vi "Read.vi"(8 "error in (no error)":errorcluster, 11 "DAQmx AI in":refnum<class "DAQmx AI.lvclass">) -> (0 "error out":errorcluster, 2 "Output":variant, 3 "DAQmx AI out":refnum<class "DAQmx AI.lvclass">)   [LabVIEW 2017, in "DAQmx AI.lvclass"]
uses:
  DAQmx AI.lvclass
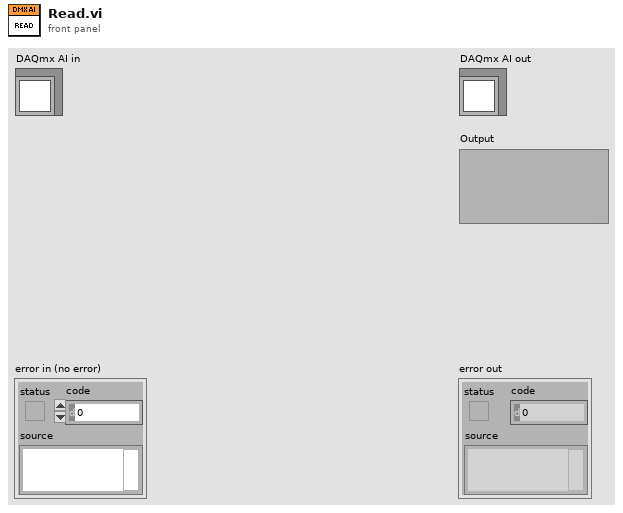
[diagram p1: front panel]
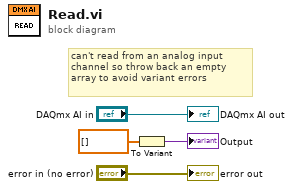
[diagram p0: block diagram]
diagram:
  # "can't read from an analog input channel so throw back an empty array to avoid variant errors"
  n1 = To Variant(anything=dbl[] []) -> (Variant=→"Output":variant)
  "error out" <- "error in (no error)"
  "DAQmx AI out" <- "DAQmx AI in"
